vi "2dgaussian001.vi"(1 "Paramters":dbl[](array[numeric]) format="%.2f") -> (0 "Flattened Image":dbl[](array[numeric]) format="%.2f")   [LabVIEW 2009]
uses:
  <vilib>/Analysis/baseanly.llb/Real Outer Product.vi
  <vilib>/Analysis/NI_AALBase.lvlib
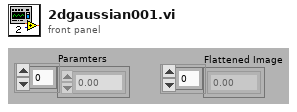
[diagram p1: front panel]
types:
  T1 = typedef "NI_Matrix.lvlib/RealMatrix.ctl" = dbl[][]
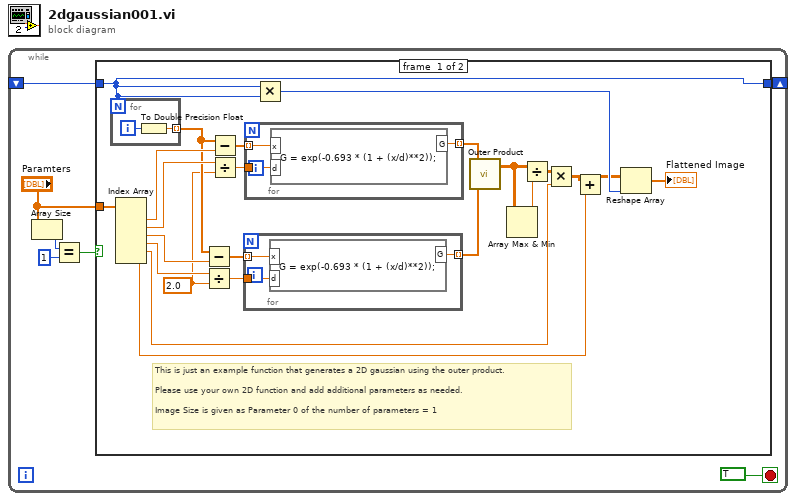
[diagram p0: block diagram]
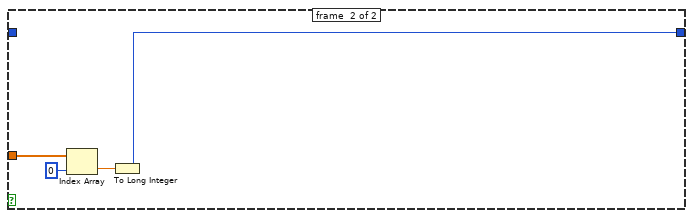
[diagram p2: hidden frame]
diagram:
  n1 = while {
    shift-right: [w1] -> _
    shift-left: _ -> [w4]
    stop <- TRUE stop-if-true
    n2 = Array Size(array="Paramters") -> (size(s)=w6:i32)
    n3 = Equal?(x=w6, y=1) -> (x = y?=w2:bool)
    n4 = case shown="False" w2 {
      tunnel: "Paramters" -> [w9 w42]
      tunnel: w4 -> [w8 _]
      tunnel: [w8 w39] -> w1
      frame #0 {
        w13 = 2.0 ("y")
        # "This is just an example function that generates a 2D gaussian using the outer product.\n\nPlease use your own 2D function and add additional parameters as needed.\n\nImage Size is given as Parameter 0 of the number of parameters = 1"
        n5 = for {
          N: w8 -> [_]
          tunnel: [w31] -> w16 mode=indexing
          i -> [w32]
          n6 = To Double Precision Float(number=w32) -> (double precision float=w31:dbl)
        }
        n7 = Index Array(array=w9) -> (element #1=w26:dbl, element #2=w27:dbl, element #3=w28:dbl, element #4=w29:dbl, element #5=w30:dbl, element #6=w10:dbl)  [unwired: 6 in]
        n8 = Subtract(x=w16, y=w28) -> (x-y=w19:dbl[])
        n9 = Divide(x=w29, y=w13) -> (x/y=w15:dbl)
        n10 = Subtract(x=w16, y=w26) -> (x-y=w20:dbl[])
        n11 = Divide(x=w27, y=w13) -> (x/y=w14:dbl)
        n12 = for {
          tunnel: [w38] -> w22 mode=indexing
          tunnel: w19 -> [w37] mode=indexing
          tunnel: w15 -> [w36]
          n13 = formula code="G = exp(-0.693 * (1 + (x/d)**2));"("x"=w37, "d"=w36) -> ("G"=w38:dbl)
        }
        n14 = for {
          tunnel: [w35] -> w21 mode=indexing
          tunnel: w20 -> [w34] mode=indexing
          tunnel: w14 -> [w33]
          n15 = formula code="G = exp(-0.693 * (1 + (x/d)**2));"("x"=w34, "d"=w33) -> ("G"=w35:dbl)
        }
        n16 = Multiply(x=w8, y=w8) -> (x*y=w17:i32)
        n17 = call-poly <vilib>:"Outer Product.vi"("Y Vector"=w22, "X Vector"=w21) -> ("Outer Product"=w24:T1)  [unwired: 1 out]
        n18 = Array Max & Min(array=w24) -> (max value=w25:dbl)  [unwired: 3 out]
        n19 = Divide(x=w24, y=w25) -> (x/y=w23:T1)
        n20 = Multiply(x=w23, y=w30) -> (x*y=w12:T1)
        n21 = Add(x=w12, y=w10) -> (x+y=w11:T1)
        n22 = Reshape Array(w11, w17) -> (→"Flattened Image":dbl[])
      }
      frame #1 {
        n23 = Index Array(array=w42, index=0) -> (element=w40:dbl)
        n24 = To Long Integer(number=w40) -> (32bit integer=w39:i32)
      }
    }
  }
